vi "Homework1.vi"() -> ()   [LabVIEW 2017]
panel:
  in  "Array 6":dbl[][](array[numeric])=[[6.0, 6.0, 6.0], [6.0, 6.0, 6.0], [6.0, 6.0, 6.0], [6.0, 6.0, 6.0]]
  out "output2":dbl[][](array[numeric])
  in  "6":bool
  in  "5":bool
  in  "4":bool
  in  "Array 5":dbl[][](array[numeric])=[[5.0, 5.0, 5.0], [5.0, 5.0, 5.0], [5.0, 5.0, 5.0], [5.0, 5.0, 5.0]]
  in  "Array 4":dbl[][](array[numeric])=[[4.0, 4.0, 4.0], [4.0, 4.0, 4.0], [4.0, 4.0, 4.0], [4.0, 4.0, 4.0]]
  in  "stop":bool
  out "output1":dbl[][](array[numeric])=[[2.0, 2.0, 2.0], [2.0, 2.0, 2.0], [2.0, 2.0, 2.0], [2.0, 2.0, 2.0]]
  in  "Combo Box":string(combo)="2"
  in  "Array 3":dbl[][](array[numeric])=[[3.0, 3.0, 3.0], [3.0, 3.0, 3.0], [3.0, 3.0, 3.0], [3.0, 3.0, 3.0]]
  in  "Array 2":dbl[][](array[numeric])=[[2.0, 2.0, 2.0], [2.0, 2.0, 2.0], [2.0, 2.0, 2.0], [2.0, 2.0, 2.0]]
  in  "Array1":dbl[][](array[numeric])=[[1.0, 1.0, 1.0], [1.0, 1.0, 1.0], [1.0, 1.0, 1.0], [1.0, 1.0, 1.0]]
  # "design with cmbobox"
  # "design with buttons"
  # "please press just one key"
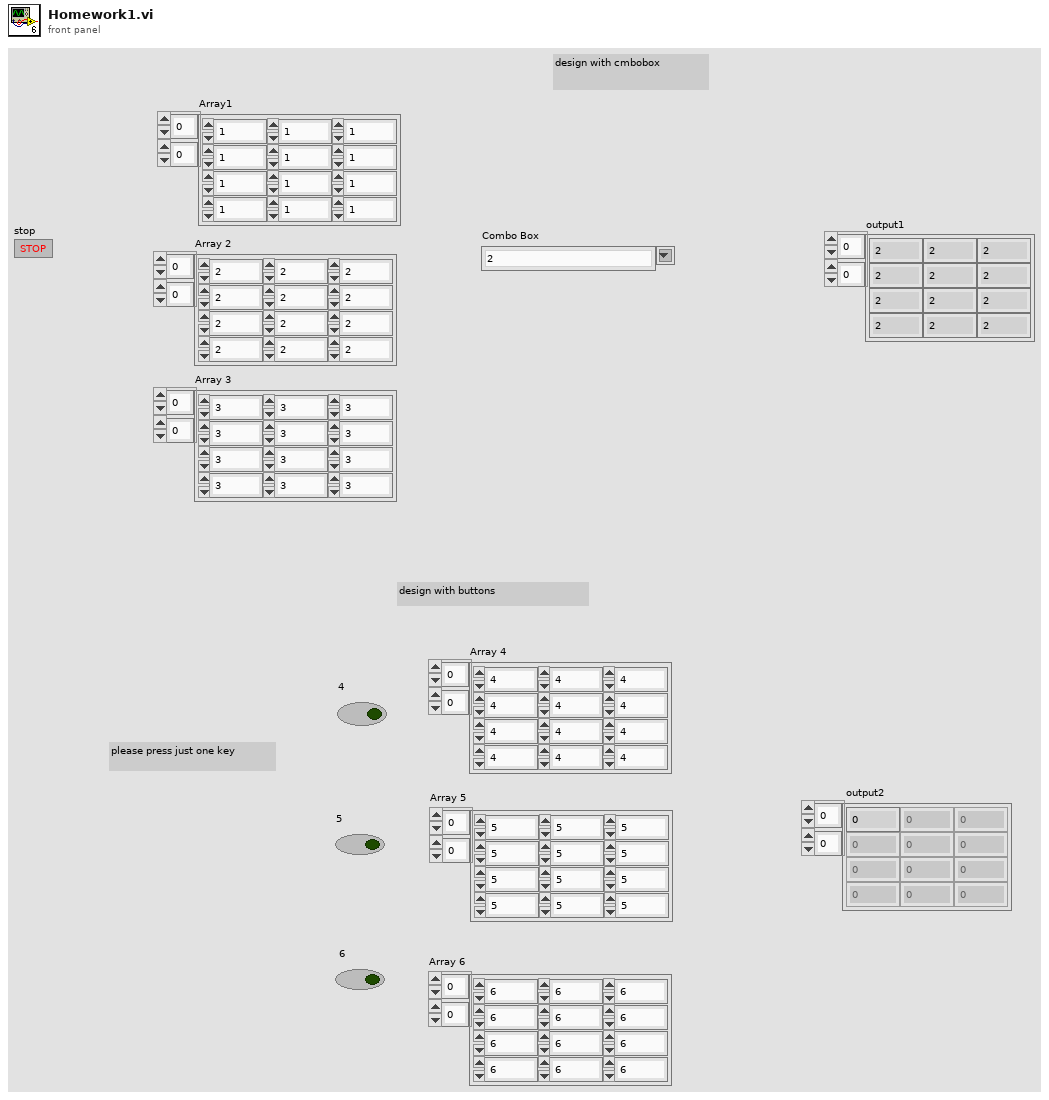
[diagram p1: front panel]
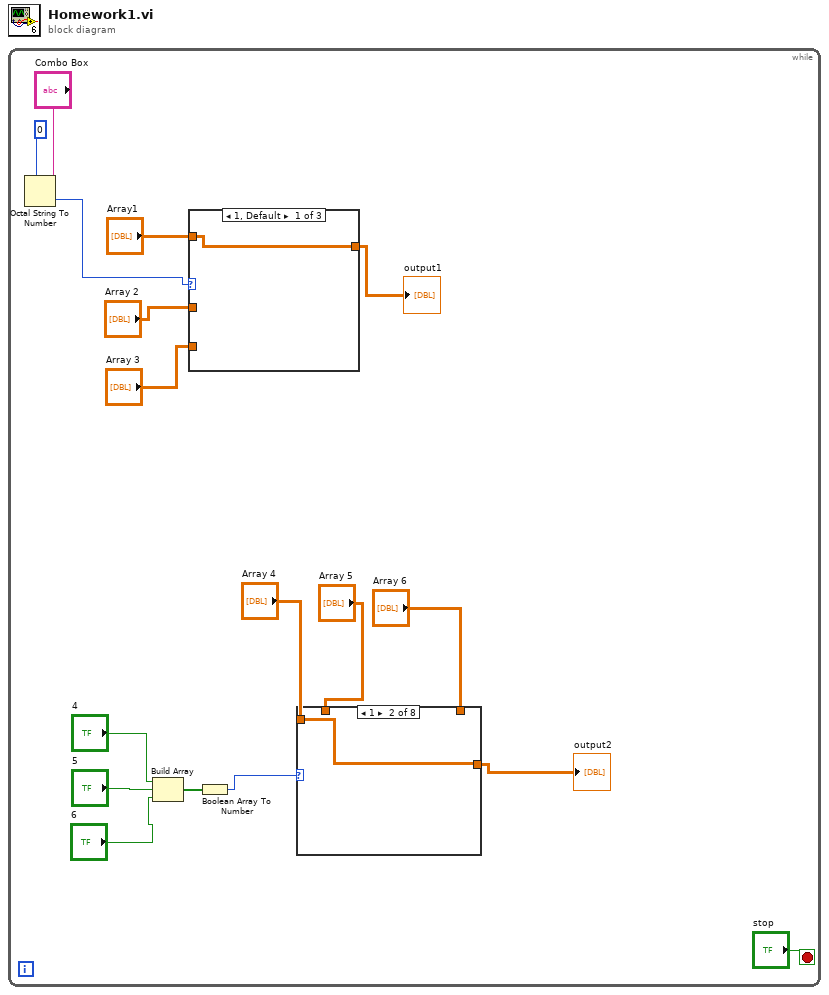
[diagram p0: block diagram]
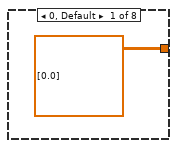
[diagram p2: hidden frame]
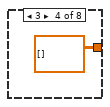
[diagram p4: hidden frame]
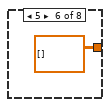
[diagram p6: hidden frame]
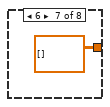
[diagram p7: hidden frame]
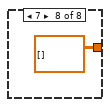
[diagram p8: hidden frame]
diagram:
  n1 = while {
    stop <- "stop" stop-if-true
    n2 = Octal String To Number(3:0 ("offset"), 4:"Combo Box") -> (0:w10:u32)  [unwired: 1 in, 1 out]
    n3 = Build Array("4", "5", "6") -> (w6:bool[])
    n4 = case shown="1, Default" w10 {
      tunnel: "Array1" -> [w26 _ _]
      tunnel: [w26 w27 w28] -> w16
      tunnel: "Array 2" -> [_ w27 _]
      tunnel: "Array 3" -> [_ _ w28]
      frame 1, Default {
      }
      frame 2 {
      }
      frame 3 {
      }
    }
    "output1" <- w16
    n5 = Boolean Array To Number(Boolean array=w6) -> (number=w5:u32)
    n6 = case shown="1" w5 {
      tunnel: "Array 4" -> [_ w19 _ _ _ _ _ _]
      tunnel: [dbl[][] [[0.0]] ("Array 7") w19 w20 dbl[][] [] ("Array 9") w22 dbl[][] [] ("Array 9") dbl[][] [] ("Array 9") dbl[][] [] ("Array 9")] -> w3
      tunnel: "Array 5" -> [_ _ w20 _ _ _ _ _]
      tunnel: "Array 6" -> [_ _ _ _ w22 _ _ _]
      frame 0, Default {
      }
      frame 1 {
      }
      frame 2 {
      }
      frame 3 {
      }
      frame 4 {
      }
      frame 5 {
      }
      frame 6 {
      }
      frame 7 {
      }
    }
    "output2" <- w3
  }
